vi "RFswitch.vi"() -> ()   [LabVIEW 2013]
uses:
  Global 1.vi
panel:
  in  "RF Channel":u32=4 min=1 max=4 step=1
  out "Bytes Written 6":i32=5
  out "Bytes Read 6":i32
  out "Read Array 6":i32[](array[numeric])
  out "Write Array 6":i32[](array[numeric])=[5, 53, 6, 0, 0]
  out "Bytes Written 7":i32=5
  out "Bytes Read 7":i32
  out "Read Array 7":i32[](array[numeric])
  out "Write Array 7":i32[](array[numeric])=[5, 53, 7, 0, 0]
  out "Handle":u32=241743216
  out "Device Description":string
  in  "Device Index":u32
  # "RF switch control panel"
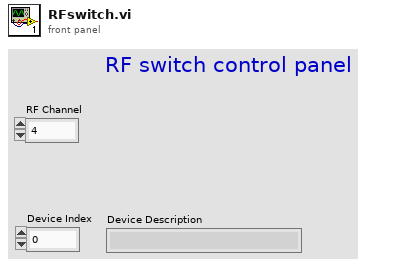
[diagram p1: front panel]
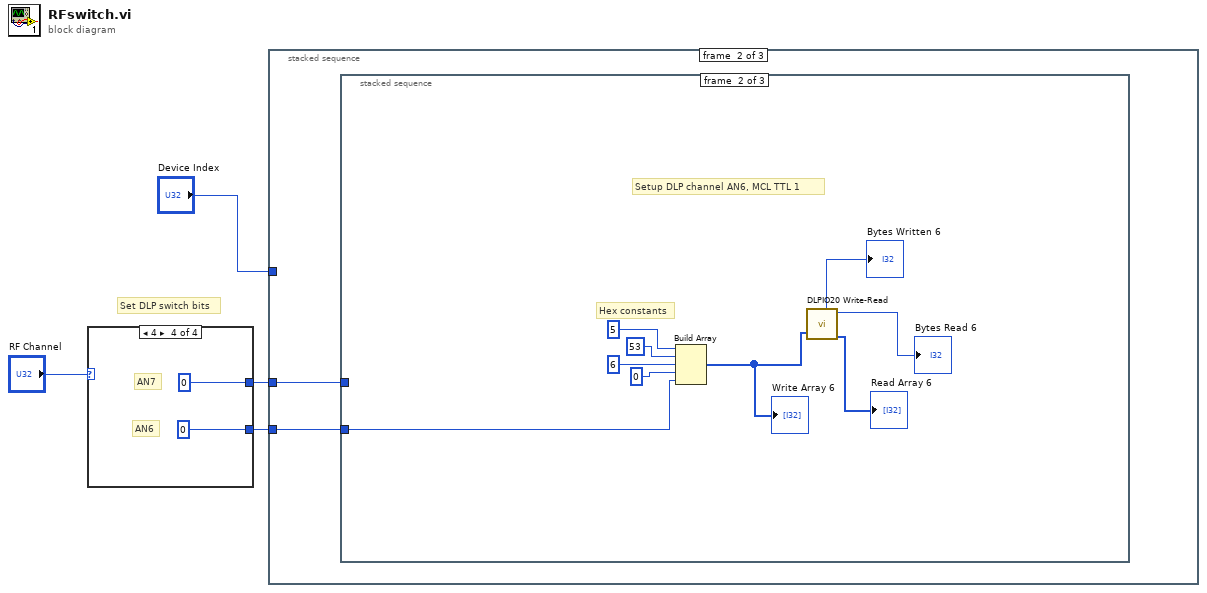
[diagram p0: block diagram]
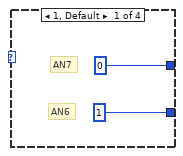
[diagram p2: hidden frame]
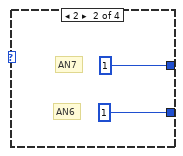
[diagram p3: hidden frame]
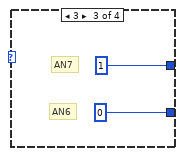
[diagram p4: hidden frame]
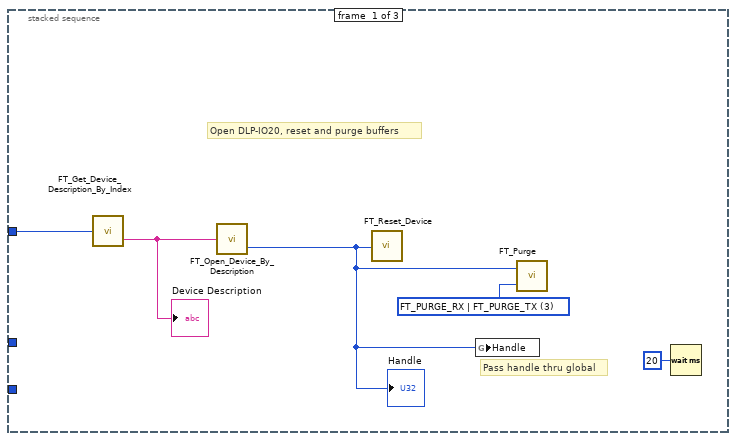
[diagram p5: hidden frame]
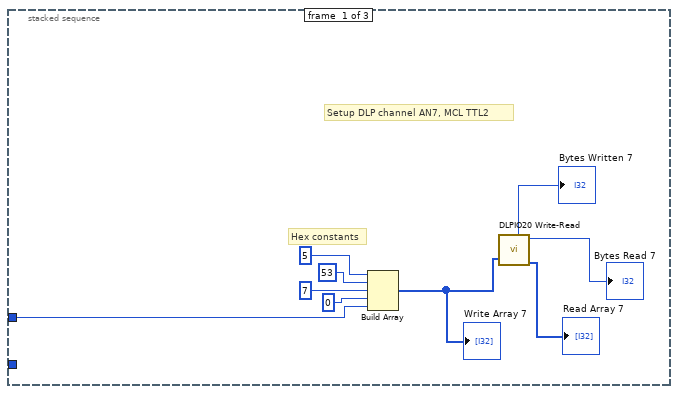
[diagram p6: hidden frame]
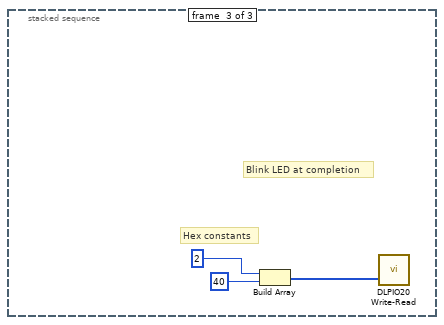
[diagram p7: hidden frame]
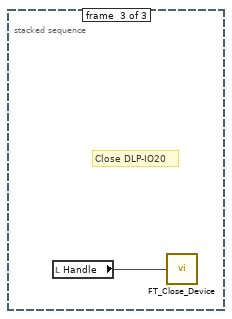
[diagram p8: hidden frame]
diagram:
  # "Set DLP switch bits"
  n1 = case shown="4" "RF Channel" {
    tunnel: [0 1 1 0] -> w2
    tunnel: [1 1 0 0] -> w1
    frame 1, Default {
      # "AN6"
      # "AN7"
    }
    frame 2 {
      # "AN6"
      # "AN7"
    }
    frame 3 {
      # "AN6"
      # "AN7"
    }
    frame 4 {
      # "AN6"
      # "AN7"
    }
  }
  n2 = stacked-sequence {
    tunnel: "Device Index" -> [w13 _ _]
    tunnel: w2 -> [_ w19 _]
    tunnel: w1 -> [_ w18 _]
    frame #0 {
      w16 = u32 3 items=["FT_PURGE_RX"=1, "FT_PURGE_TX"=2, "FT_PURGE_RX | FT_PURGE_TX"=3] ("Purge Flags")
      # "Pass handle thru global"
      # "Open DLP-IO20, reset and purge buffers"
      n3 = call "FT_Get_Device_Description_By_Index.vi"("Device Index"=w13) -> ("Device Description"=w17:string)  [unwired: 1 out]
      "Device Description" <- w17
      n4 = call "FT_Open_Device_By_Description.vi"("Device Description"=w17) -> ("Handle"=w14:u32)  [unwired: 1 out]
      "Handle" <- w14
      n5 = call "FT_Reset_Device.vi"("Handle"=w14) -> ()  [unwired: 1 out]
      n6 = global write "Global 1.vi" "Handle"(w14) -> ()
      n7 = call "FT_Purge.vi"("Purge Flags"=w16, "Handle"=w14) -> ()  [unwired: 1 out]
      n8 = Wait (ms)(milliseconds to wait=u32 20) -> ()  [unwired: 1 out]
    }
    frame #1 {
      n9 = stacked-sequence {
        tunnel: w19 -> [w20 _ _]
        tunnel: w18 -> [_ w29 _]
        frame #0 {
          # "Setup DLP channel AN7, MCL TTL2"
          # "Hex constants"
          n10 = Build Array "Build Array"(u8 5, u8 53, u8 7, u8 0, w20) -> (w23:i32[])
          "Write Array 7" <- w23
          n11 = call "DLPIO20 Write-Read.vi"("Write Buffer"=w23) -> ("Read Buffer Out"=→"Read Array 7":u8[], "Bytes Read"=→"Bytes Read 7":u32, "Bytes Written"=→"Bytes Written 7":u32)  [unwired: 3 in]
        }
        frame #1 {
          # "Setup DLP channel AN6, MCL TTL 1"
          # "Hex constants"
          n12 = Build Array "Build Array"(u8 5, u8 53, u8 6, u8 0, w29) -> (w32:i32[])
          "Write Array 6" <- w32
          n13 = call "DLPIO20 Write-Read.vi"("Write Buffer"=w32) -> ("Read Buffer Out"=→"Read Array 6":u8[], "Bytes Read"=→"Bytes Read 6":u32, "Bytes Written"=→"Bytes Written 6":u32)  [unwired: 3 in]
        }
        frame #2 {
          # "Blink LED at completion"
          # "Hex constants"
          n14 = Build Array "Build Array"(u8 2, u8 40) -> (w38:u8[])
          n15 = call "DLPIO20 Write-Read.vi"("Write Buffer"=w38) -> ()  [unwired: 3 in, 3 out]
        }
      }
    }
    frame #2 {
      # "Close DLP-IO20"
      n16 = local read "Handle"() -> (w41:u32)
      n17 = call "FT_Close_Device.vi"("Handle"=w41) -> ()  [unwired: 1 out]
    }
  }
